vi "Set Process UEs.vi"(10 "Process UEs":refnum<user-event>[](array[refnum]), 11 "Process in":refnum<class "Process.lvclass">) -> (3 "Process out":refnum<class "Process.lvclass">)   [LabVIEW 2019, in "TelemetryAsync Engine.lvlib" / "Process.lvclass"]
uses:
  Process.lvclass
  TypeDefs/Update.ctl
  Process.lvclass/Process.ctl
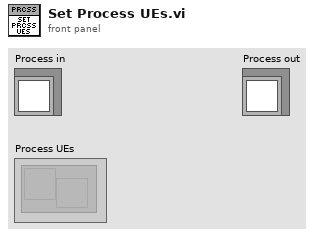
[diagram p1: front panel]
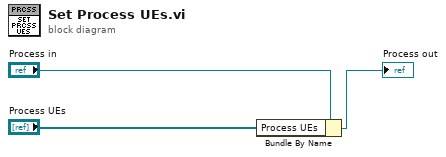
[diagram p0: block diagram]
diagram:
  n1 = Bundle By Name(cluster="Process in", "Process UEs"="Process UEs") -> (→"Process out":refnum<class "Process.lvclass">)
